vi "Swerve Drive.vi"(0 "X":dbl(slide) scale=-1.0..1.0, 1 "Rot. Point Y":dbl, 3 "Rot. Point X":dbl, 7 "Y":dbl(slide) scale=1.0..-1.0, 11 "Z":dbl(knob) scale=1.0..-1.0, 12 "Auto Controls":bool, 13 "Robot-Centric":bool) -> ()   [LabVIEW 2016]
panel:
  in  "Robot Length":dbl=21.5
  in  "Robot Width":dbl=29.5
  # "SWERVE DRIVE\nVersion 3.1\n\nCory Lynch\nApple Pi Robotics\nTeam 2067"
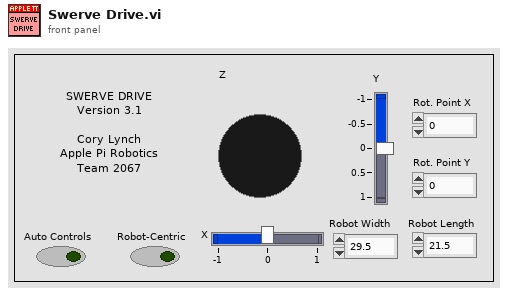
[diagram p1: front panel]
types:
  T1 = enum16{"Back Left", "Back Right", "Front Left", "Front Right"}
  T2 = typedef "WPI_MotorControlDeviceRef.ctl" = cluster{"DeviceStatus":errorcluster, "Type":T3, "PWM":cluster{"PWM Channel":T4, "DeadBand":T5}, "CAN":cluster{"Device Number":u8, "SetOutput VI Ref":variant, "GetOutput VI Ref":variant, "Enable VI Ref":variant, "Disable VI Ref":variant, "Data":variant}, "Invert":bool}
  T3 = typedef "WPI_MotorControlType.ctl" = enum16{"PWM", "CAN"}
  T4 = typedef "FPGA_DIOPWMChannel.ctl" = enum8{"PWM 0", "PWM 1", "PWM 2", "PWM 3", "PWM 4", "PWM 5", "PWM 6", "PWM 7", "PWM 8", "PWM 9", "PWM MXP 0", "PWM MXP 1", "PWM MXP 2", "PWM MXP 3", "PWM MXP 4", "PWM MXP 5", "PWM MXP 6", "PWM MXP 7", "PWM MXP 8", "PWM MXP 9", "Invalid"}
  T5 = typedef "WPI_PWMDeadband.ctl" = cluster{"Name":string, "maxPositivePwm":i32, "minPositivePwm":i32, "centerPwm":i32, "maxNegativePwm":i32, "minNegativePwm":i32, "angularRange":u16}
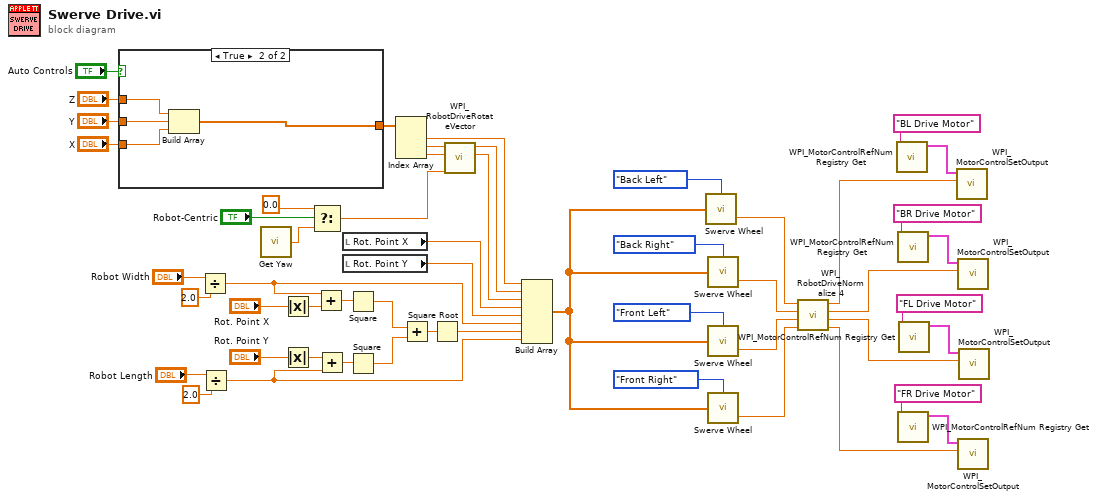
[diagram p0: block diagram]
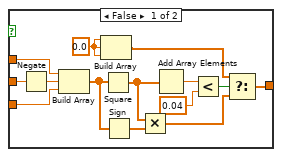
[diagram p2: hidden frame]
diagram:
  n1 = case shown="True" "Auto Controls" {
    tunnel: "Y" -> [w64 w70]
    tunnel: "X" -> [w58 w71]
    tunnel: "Z" -> [w54 w68]
    tunnel: [w55 w69] -> w10
    frame False {
      w62 = 0.0 ("element")
      n2 = Negate(x=w64) -> (-x=w57:dbl)
      n3 = Build Array(w54, w57, w58) -> (w61:dbl[])
      n4 = Build Array(w62, w62, w62) -> (w63:dbl[])
      n5 = Square(x=w61) -> (x^2=w59:dbl[])
      n6 = Sign(1:w61) -> (0:w60:dbl[])
      n7 = Multiply(x=w59, y=w60) -> (x*y=w56:dbl[])
      n8 = Add Array Elements(numeric array=w59) -> (sum=w67:dbl)
      n9 = Less?(x=w67, y=0.04 ("x")) -> (x < y?=w65:bool)
      n10 = Select(t=w63, s=w65, f=w56) -> (s? t:f=w55:dbl[])
    }
    frame True {
      n11 = Build Array(w68, w70, w71) -> (w69:dbl[])
    }
  }
  n12 = Divide(x="Robot Width", y=2.0) -> (x/y=w14:dbl)
  n13 = Divide(x="Robot Length", y=2.0) -> (x/y=w12:dbl)
  n14 = call "Get Yaw.vi"() -> ("Angle"=w1:dbl)  [unwired: 1 in]
  n15 = Absolute Value(x="Rot. Point X") -> (abs(x)=w32:dbl)
  n16 = Absolute Value(x="Rot. Point Y") -> (abs(x)=w30:dbl)
  n17 = Select(t=0.0, s="Robot-Centric", f=w1) -> (s? t:f=w5:dbl)
  n18 = Add(x=w14, y=w32) -> (x+y=w31:dbl)
  n19 = Add(x=w30, y=w12) -> (x+y=w29:dbl)
  n20 = local read "Rot. Point X"() -> (w16:dbl)
  n21 = local read "Rot. Point Y"() -> (w15:dbl)
  n22 = Square(x=w31) -> (x^2=w27:dbl)
  n23 = Square(x=w29) -> (x^2=w28:dbl)
  n24 = Index Array(array=w10) -> (element #1=w4:dbl, element #2=w11:dbl, element #3=w19:dbl)  [unwired: 3 in]
  n25 = Add(x=w27, y=w28) -> (x+y=w26:dbl)
  n26 = Square Root(x=w26) -> (sqrt(x)=w13:dbl)
  n27 = call <vilib>:"WPI_RobotDriveRotateVector.vi"("Angle"=w5, "X"=w19, "Y"=w11) -> ("X'"=w8:dbl, "Y'"=w3:dbl)  [unwired: 7 out]
  n28 = Build Array(w4, w3, w8, w16, w15, w14, w13, w12) -> (w9:dbl[])
  n29 = call "Swerve Wheel.vi"("Wheel"=T1."Back Left", "Inputs"=w9) -> ("Speed"=w50:dbl)  [unwired: 3 in]
  n30 = call "Swerve Wheel.vi"("Wheel"=T1."Back Right", "Inputs"=w9) -> ("Speed"=w49:dbl)  [unwired: 3 in]
  n31 = call "Swerve Wheel.vi"("Wheel"=T1."Front Left", "Inputs"=w9) -> ("Speed"=w48:dbl)  [unwired: 3 in]
  n32 = call "Swerve Wheel.vi"("Wheel"=T1."Front Right", "Inputs"=w9) -> ("Speed"=w47:dbl)  [unwired: 3 in]
  n33 = call <vilib>:"WPI_RobotDriveNormalize 4.vi"("D"=w47, "C"=w48, "B"=w49, "A"=w50) -> ("D'"=w34:dbl, "C'"=w35:dbl, "B'"=w36:dbl, "A'"=w37:dbl)
  n34 = call <vilib>:"WPI_MotorControlRefNum Registry Get.vi"("refnum name"="BL Drive Motor") -> ("MotorControlDevRef"=w45:T2)  [unwired: 9 in, 1 out]
  n35 = call <vilib>:"WPI_MotorControlRefNum Registry Get.vi"("refnum name"="BR Drive Motor") -> ("MotorControlDevRef"=w42:T2)  [unwired: 9 in, 1 out]
  n36 = call <vilib>:"WPI_MotorControlRefNum Registry Get.vi"("refnum name"="FR Drive Motor") -> ("MotorControlDevRef"=w38:T2)  [unwired: 9 in, 1 out]
  n37 = call <vilib>:"WPI_MotorControlRefNum Registry Get.vi"("refnum name"="FL Drive Motor") -> ("MotorControlDevRef"=w41:T2)  [unwired: 9 in, 1 out]
  n38 = call <vilib>:"WPI_MotorControlSetOutput.vi"("Output"=w37, "MotorControlDevRef"=w45) -> ()  [unwired: 7 in, 3 out]
  n39 = call <vilib>:"WPI_MotorControlSetOutput.vi"("Output"=w36, "MotorControlDevRef"=w42) -> ()  [unwired: 7 in, 3 out]
  n40 = call <vilib>:"WPI_MotorControlSetOutput.vi"("Output"=w34, "MotorControlDevRef"=w38) -> ()  [unwired: 7 in, 3 out]
  n41 = call <vilib>:"WPI_MotorControlSetOutput.vi"("Output"=w35, "MotorControlDevRef"=w41) -> ()  [unwired: 7 in, 3 out]
